vi "gen_digital_on_off.vi"(7 "sampling rate":dbl format="%#_6p", 8 "waveform length":i32, 11 "On / Off":bool) -> (3 "digital waveform":digitalwaveform(waveform)={"t0"=timestamp(0 s since 1904-01-01), "dt"=0.0, "Y"={"transitions"=[], "data"=[]}, "error"={"status"=FALSE, "code"=37421928, "source"=""}})   [LabVIEW 2019]
uses:
  <vilib>/Waveform/DWDTOps.llb/DWDT Analog to Digital.vi
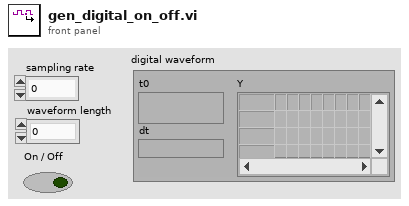
[diagram p1: front panel]
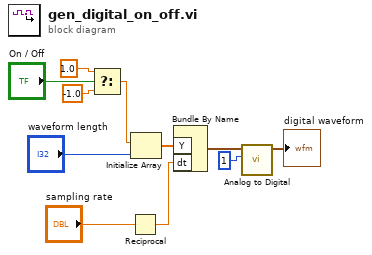
[diagram p0: block diagram]
diagram:
  n1 = Select(t=1.0, s="On / Off", f=-1.0) -> (s? t:f=w7:dbl)
  n2 = Reciprocal(x="sampling rate") -> (1/x=w5:dbl)
  n3 = Initialize Array(w7, "waveform length") -> (w3:dbl[])
  n4 = Bundle By Name("Y"=w3, "dt"=w5) -> (w6:waveform(dbl))  [unwired: 1 in]
  n5 = call-poly <vilib>:"Analog to Digital.vi"("resolution (16 bit)"=1, "analog waveform"=w6) -> ("digital waveform"=→"digital waveform":digitalwaveform)  [unwired: 6 in, 3 out]
